vi "Recording test.vi"() -> ()   [LabVIEW 2015]
uses:
  <resource>/objmgr/daqmx.rc
panel:
  in  "SampQuant.SampPerChan":dbl
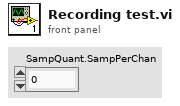
[diagram p1: front panel]
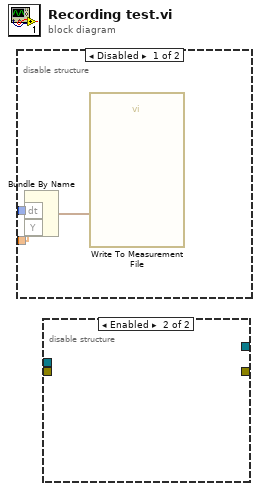
[diagram p0: block diagram]
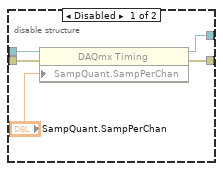
[diagram p2: hidden frame]
diagram:
  n1 = disable-structure shown="Disabled" {
    disable-tunnel: _ -> [w2 _]
    disable-tunnel: _ -> [w1 _]
    frame Disabled {
      n2 = Bundle By Name("dt"=w1, "Y"=w2) -> (w3:waveform(dbl))  [unwired: 1 in]
      n3 = call "Write To Measurement File"("Signals"=w3) -> ()  [unwired: 16 in, 3 out]
    }
    frame Enabled {
    }
  }
  n4 = disable-structure shown="Enabled" {
    disable-tunnel: _ -> [w8 _]
    disable-tunnel: _ -> [w7 _]
    disable-tunnel: [w5 _] -> _
    disable-tunnel: [w4 _] -> _
    frame Disabled {
      n5 = property class="DAQmx Timing"(reference=w7, error in=w8, "SampQuant.SampPerChan"="SampQuant.SampPerChan") -> (reference out=w4:refnum<k21>, error out=w5:errorcluster)
    }
    frame Enabled {
    }
  }
